vi "LaunchManualMode.vi"(8 "error in (no error)":errorcluster, 11 "MainData":T1) -> (0 "error out":errorcluster, 3 "MainData out":T1)   [LabVIEW 2019, in "MainController.lvlib"]
uses:
  MainController.lvlib
  Cluster - MainData.ctl
  All Message Queues.ctl
  Cluster - MainControllerMessage.ctl
  Enum - MainState.ctl
  AutoMode/Cluster - AutoModeMessage.ctl
  AutoMode/Enum - AutoModeState.ctl
  ManualMode/Cluster - ManualModeMessageCluster.ctl
  ManualMode/Enum - ManualModeMessage.ctl
  Settings/CTL_MessageCluster.ctl
  Settings/CTL_SettingsMessage.ctl
  Cluster - HardwareConfiguration.ctl
  Cluster - LoggingConfiguration.ctl
  Cluster - TestSettings.ctl
  UI State.ctl
  UI Data.ctl
  ManualMode/ManualMode.vi
  support/User Interface/UserInterface.lvlib
  ManualMode/ManualMode.lvlib
  AutoMode/AutoMode.lvlib
  Settings/Settings.lvlib
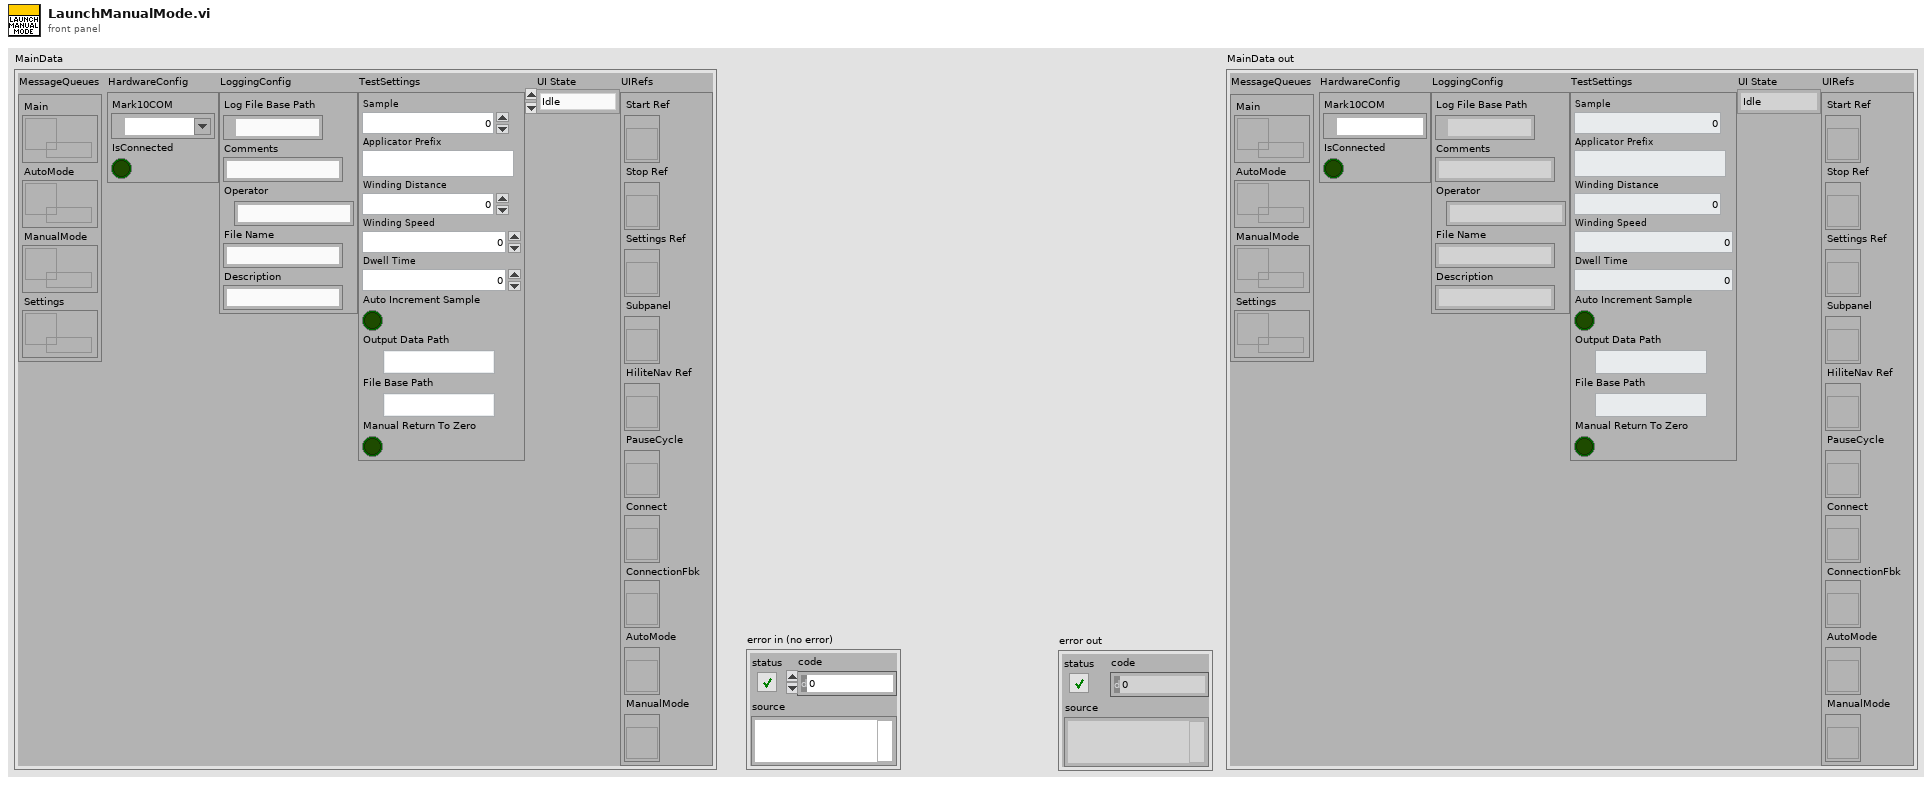
[diagram p1: front panel]
types:
  T1 = typedef "MainController.lvlib/Cluster - MainData.ctl" = cluster{"MessageQueues":T2, "HardwareConfig":T3, "LoggingConfig":T4, "TestSettings":T5, "UI State":T6, "UIRefs":T7}
  T2 = typedef "MainController.lvlib/All Message Queues.ctl" = cluster{"Main":refnum<queue>, "AutoMode":refnum<queue>, "ManualMode":refnum<queue>, "Settings":refnum<queue>}
  T3 = typedef "MainController.lvlib/Cluster - HardwareConfiguration.ctl" = cluster{"Mark10COM":refnum<visa-resource-name>, "IsConnected":bool}
  T4 = typedef "MainController.lvlib/Cluster - LoggingConfiguration.ctl" = cluster{"Log File Base Path":path, "Comments ":string, "Operator":string, "File Name":string, "Description":string}
  T5 = typedef "MainController.lvlib/Cluster - TestSettings.ctl" = cluster{"Sample":u32, "Applicator Prefix":string, "Winding Distance":dbl, "Winding Speed":dbl, "Dwell Time":dbl, "Auto Increment Sample":bool, "Output Data Path":path, "File Base Path":path, "Manual Return To Zero":bool}
  T6 = typedef "MainController.lvlib/UI State.ctl" = enum16{"Idle", "AutoIdle", "AutoRunning", "ManualMode", "Settings"}
  T7 = typedef "MainController.lvlib/UI Data.ctl" = cluster{"Start Ref":refnum<vi>, "Stop Ref":refnum<vi>, "Settings Ref":refnum<vi>, "Subpanel":refnum<vi>, "HiliteNav Ref":refnum<vi>, "PauseCycle":refnum<vi>, "Connect":refnum<vi>, "ConnectionFbk":refnum<vi>, "AutoMode":refnum<vi>, "ManualMode":refnum<vi>}
  T8 = typedef "MainController.lvlib/Enum - MainState.ctl" = enum16{"Initialize", "InitUIRefs", "LaunchSettings", "LaunchAutoMode", "LaunchManualMode", "LaunchTestReport", "ConnectHardware", "DisconnectHardware", "HiliteNavItems", "StartAutoMode", "PauseAutoMode", "StopAutoMode", "ShowFlyout", "HideFlyout", "BroadcastSettings", "PickupTestSettings", "BroadcastHW", "AutoTestDone", "DAQStatus", "UpdateCommandBar", "Error", "RecieveError", "Exit"}
  T9 = typedef "ManualMode.lvlib/Enum - ManualModeMessage.ctl" = enum16{"Initialize", "Idle", "Start", "Stop", "Pause", "Resume", "BroadcastPreCollection", "MoveCCW", "MoveCW", "StopMove", "SetZero", "GotoZero", "UpdateHW", "Error", "Exit"}
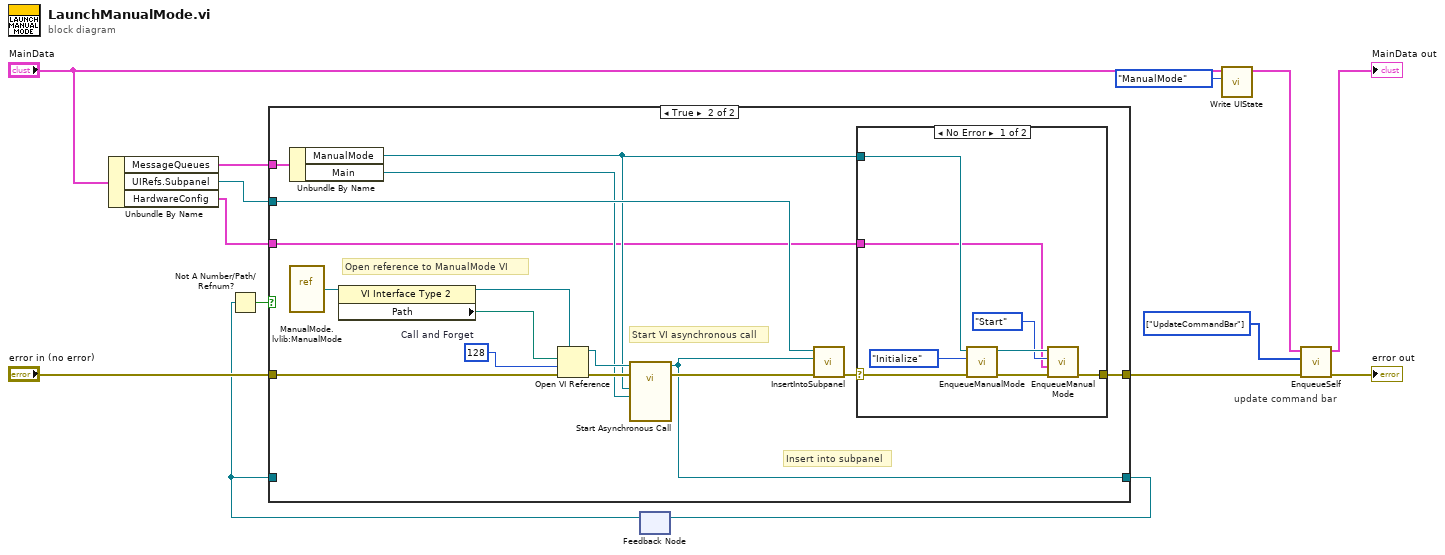
[diagram p0: block diagram]
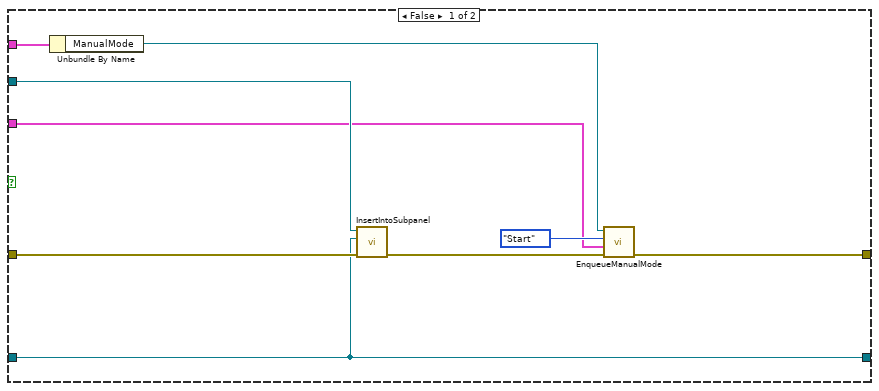
[diagram p2: hidden frame]
diagram:
  w1 = T8[] [enum."UpdateCommandBar"] items=["Initialize", "InitUIRefs", "LaunchSettings", "LaunchAutoMode", "LaunchManualMode", "LaunchTestReport", "ConnectHardware", "DisconnectHardware", "HiliteNavItems", "StartAutoMode", "PauseAutoMode", "StopAutoMode", "ShowFlyout", "HideFlyout", "BroadcastSettings", "PickupTestSettings", "BroadcastHW", "AutoTestDone", "DAQStatus", "UpdateCommandBar", "Error", "RecieveError", "Exit"] ("Messages")
  # "update command bar"
  n1 = Unbundle By Name("MainData") -> ("MessageQueues"=w9:T2, "UIRefs.Subpanel"=w8:refnum<vi>, "HardwareConfig"=w7:T3)
  n2 = feedback #1() -> (w11:refnum<vi>)  [unwired: 1 in]
  n3 = Not A Number/Path/Refnum?(number/path/refnum=w11) -> (NaN/Path/Refnum?=w10:bool)
  n4 = case shown="True" w10 {
    tunnel: "error in (no error)" -> [w23 w39]
    tunnel: w8 -> [w22 w38]
    tunnel: [w19 w34] -> w13
    tunnel: [w20 w31] -> w12
    tunnel: w11 -> [w20 _]
    tunnel: w9 -> [w18 w27]
    tunnel: w7 -> [w15 w24]
    frame False {
      n5 = Unbundle By Name(w18) -> ("ManualMode"=w17:refnum<queue>)
      n6 = call "InsertIntoSubpanel.vi"("error in (no error)"=w23, "VI Ref"=w20, "Subpanel"=w22) -> ("error out"=w21:errorcluster)  [unwired: 8 in]
      n7 = call "EnqueueManualMode.vi"("error in (no error)"=w21, "Data"=w15, "Message"=Enum_-_ManualModeMessage."Start", "queue"=w17) -> ("error out"=w19:errorcluster)  [unwired: 6 in, 1 out]
    }
    frame True {
      w33 = 128  # Call and Forget
      # "Insert into subpanel"
      # "Start VI asynchronous call"
      # "Open reference to ManualMode VI"
      n8 = Unbundle By Name(w27) -> ("ManualMode"=w25:refnum<queue>, "Main"=w26:refnum<queue>)
      n9 = vi-ref "ManualMode.lvlib:ManualMode.vi"() -> (w30:refnum<vi>)
      n10 = property class="VI Interface Type 2"(reference=w30) -> (reference out=w28:refnum<vi>, "Path"=w29:path)  [unwired: 1 in, 1 out]
      n11 = Open VI Reference(type specifier VI Refnum (for type only)=w28, vi path=w29, options=w33, error in (no error)=w39) -> (vi reference=w37:refnum<vi>, error out=w36:errorcluster)  [unwired: 2 in]
      n12 = call-by-ref "Start Asynchronous Call"(reference=w37, error in=w36, "MainUI"=w26, "ManualModeQueue"=w25) -> (reference out=w31:refnum<vi>, error out=w32:errorcluster)  [unwired: 9 in, 1 out]
      n13 = call "InsertIntoSubpanel.vi"("error in (no error)"=w32, "VI Ref"=w31, "Subpanel"=w38) -> ("error out"=w35:errorcluster)  [unwired: 8 in]
      n14 = case shown="No Error" w35 {
        selector: w35 -> [w47 w48]
        tunnel: [w41 w48] -> w34
        tunnel: w25 -> [w45 _]
        tunnel: w24 -> [w40 _]
        frame No Error {
          n15 = call "EnqueueManualMode.vi"("error in (no error)"=w47, "Message"=Enum_-_ManualModeMessage."Initialize" ("PreCollectionMessage"), "queue"=w45) -> ("error out"=w42:errorcluster, "queue out"=w44:refnum<queue>)  [unwired: 7 in]
          n16 = call "EnqueueManualMode.vi"("error in (no error)"=w42, "Data"=w40, "Message"=Enum_-_ManualModeMessage."Start", "queue"=w44) -> ("error out"=w41:errorcluster)  [unwired: 6 in, 1 out]
        }
        frame Error {
        }
      }
    }
  }
  n17 = feedback-in #1(w12) -> ()
  n18 = call "Write UIState.vi"("UI State"=UI_State."ManualMode", "MainData"="MainData") -> ("MainData out"=w2:T1)  [unwired: 9 in]
  n19 = call "EnqueueSelf.vi"("Error In"=w13, "Messages"=w1, "MainData"=w2) -> ("Error Out"=→"error out":errorcluster, "MainData out"=→"MainData out":T1)  [unwired: 7 in]
